vi "Dispose.vi"(8 "error in (no error)":errorcluster caption="错误输入（无错误）", 11 "KnownColor 输入":refnum<class "Color.lvclass"> caption="DNL_LabVIEW Object in") -> (0 "error out":errorcluster caption="错误输出")   [LabVIEW 2012, in "Color.lvclass"]
uses:
  Color.lvclass
  Color.lvclass/Color.ctl
panel:
  out "KnownColor 输出":refnum<class "Color.lvclass"> caption="DNL_LabVIEW Object out"
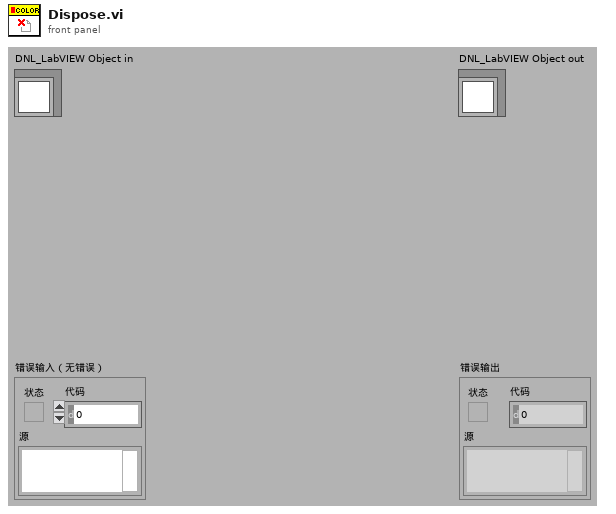
[diagram p1: front panel]
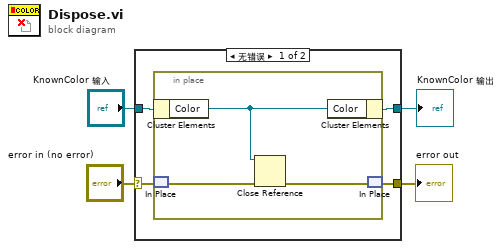
[diagram p0: block diagram]
diagram:
  n1 = case shown="无错误" "error in (no error)" {
    selector: "error in (no error)" -> [w7 w13]
    tunnel: [w6 w13] -> w3
    tunnel: [w5 w12] -> w1
    tunnel: "KnownColor 输入" -> [w8 w12]
    frame No Error {
      n2 = in-place {
        n3 = in-place-cluster #1(w8) -> ("Color"=w9:refnum<k24>)
        n4 = in-place-match #2(w7) -> (w11:errorcluster)
        n5 = Close Reference(reference=w9, error in (no error)=w11) -> (error out=w10:errorcluster)
        n6 = in-place-cluster #1("Color"=w9) -> (w5:refnum<class "Color.lvclass">)
        n7 = in-place-match #2(w10) -> (w6:errorcluster)
      }
    }
    frame Error {
    }
  }
  "error out" <- w3
  "KnownColor 输出" <- w1
